vi "Construct INI File Section Configuration.vi"(9 "Create File If Not Found? (T)":bool=TRUE, 10 "File Section":string, 11 "INI File Path":path) -> (3 "IniFileSection out":refnum<class "IniFileSection.lvclass">)   [LabVIEW 2017, in "IniFileSection.lvclass"]
uses:
  IniFileSection.lvclass
  IniFileSection.lvclass/IniFileSection.ctl
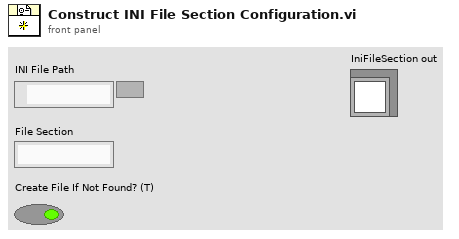
[diagram p1: front panel]
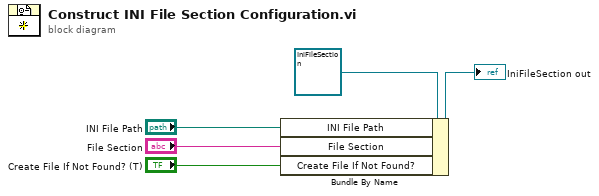
[diagram p0: block diagram]
diagram:
  n1 = Bundle By Name(cluster=refnum<class "IniFileSection.lvclass"> refnum ("IniFileSection in"), "INI File Path"="INI File Path", "File Section"="File Section", "Create File If Not Found?"="Create File If Not Found? (T)") -> (→"IniFileSection out":refnum<class "IniFileSection.lvclass">)
